vi "ConfDB-GFV.vi"(8 "error in (no error)":errorcluster, 10 "Data in":variant, 11 "Command In":T1=enum."Configure DB") -> (0 "error out":errorcluster, 2 "Data out":variant)   [LabVIEW 2013]
uses:
  ConfEnum.ctl
  ConfDB.ctl
  TypeDef/Magnification.ctl
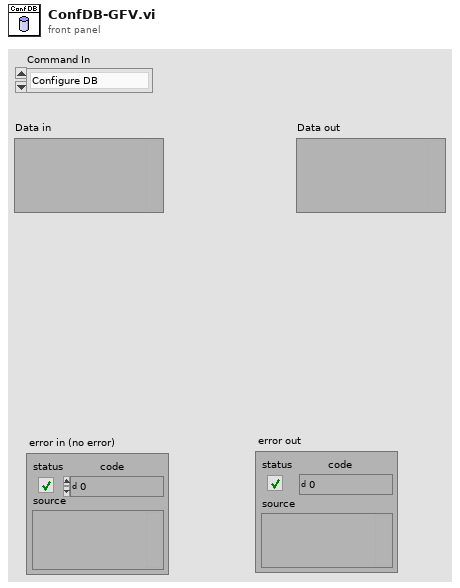
[diagram p1: front panel]
types:
  T1 = typedef "ConfEnum.ctl" = enum16{"Init", "GetConfDB", "GetTemperatureAtIndex", "WriteConfDB", "Configure DB"}
  T2 = typedef "ConfDB.ctl" = cluster{"NumberOfImages":i32, "NoImages2SaveAroundFreeze":i32, "Path":path, "NameOfPartialFile":string, "StartIndex":i32, "NumberOfStdTol":i32, "Detla t (sec)":i32, "Number of images for baseline":i32, "Temperature File Name":string, "Score":dbl, "Index number of Files":i32[], "End Index":i32, "Temperature Array":dbl[], "TStartIndex":i32, "Magnification (Microns/Pixel)":T3, "Circle Descriptor":cluster{"Min Radius":dbl, "Max Radius":dbl}}
  T3 = typedef "Magnification.ctl" = dbl
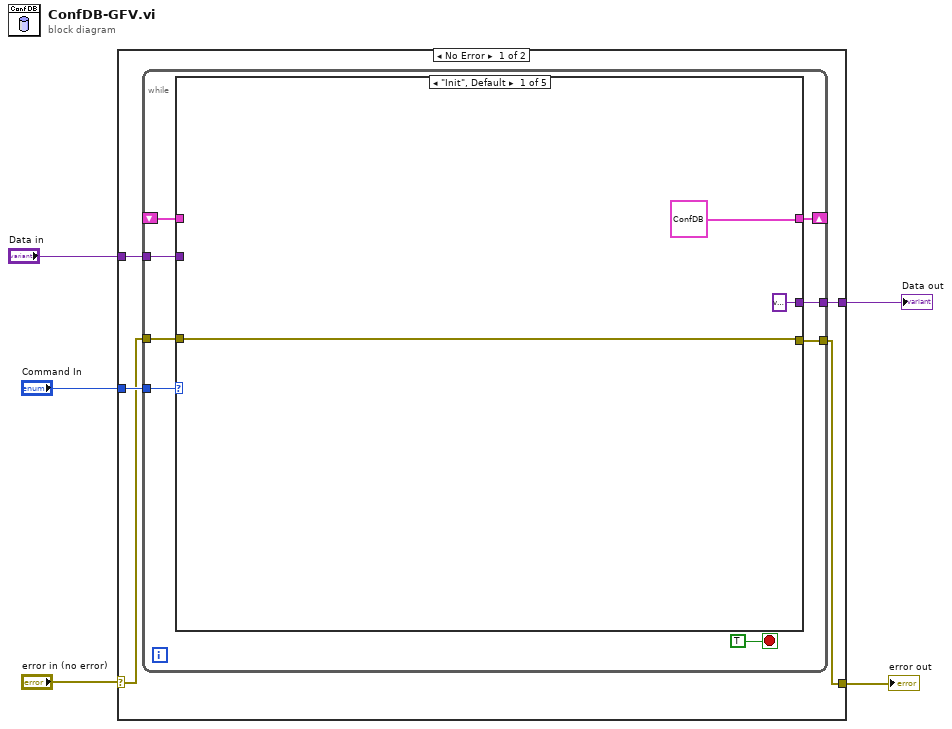
[diagram p0: block diagram]
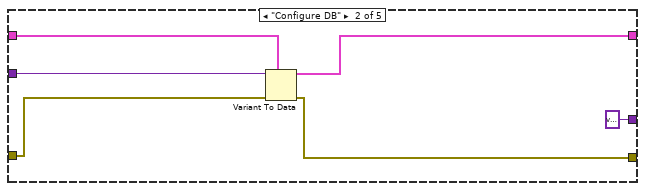
[diagram p2: hidden frame]
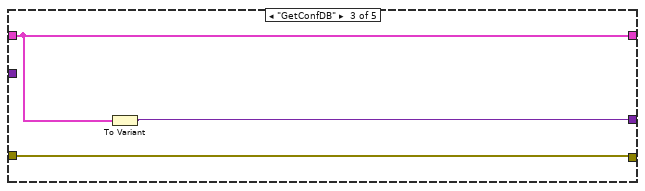
[diagram p3: hidden frame]
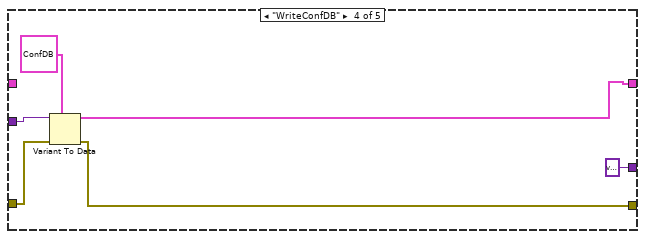
[diagram p4: hidden frame]
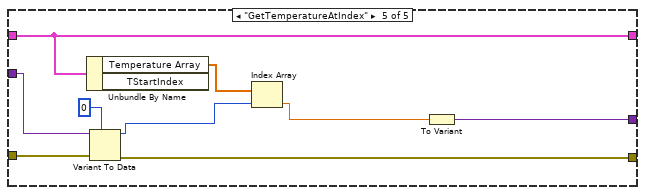
[diagram p5: hidden frame]
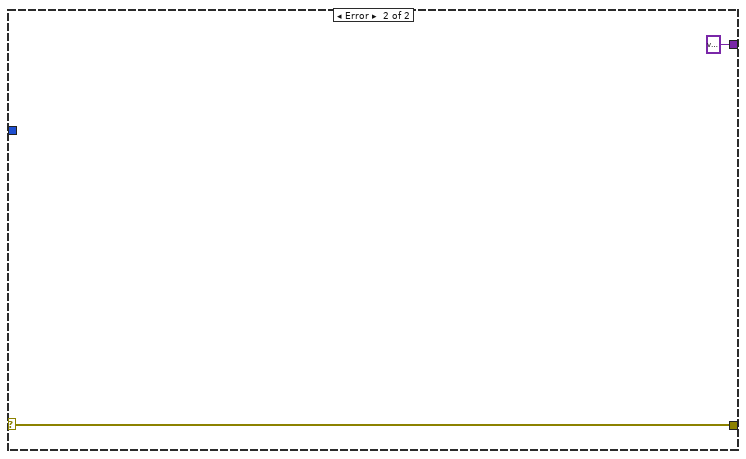
[diagram p6: hidden frame]
diagram:
  n1 = case shown="No Error" "error in (no error)" {
    selector: "error in (no error)" -> [w7 w47]
    tunnel: [w6 w47] -> w4
    tunnel: "Command In" -> [w10 _]
    tunnel: "Data in" -> [w9 _]
    tunnel: [w8 variant ("Variant")] -> w1
    frame No Error {
      n2 = while {
        tunnel: w10 -> [w17]
        shift-right: [w16] -> _
        shift-left: _ -> [w14]
        tunnel: w9 -> [w15]
        tunnel: [w13] -> w8
        tunnel: w7 -> [w12]
        tunnel: [w11] -> w6
        stop <- TRUE stop-if-true
        n3 = case shown="\"Init\", Default" w17 {
          tunnel: [T2 {"NumberOfImages"=0, "NoImages2SaveAroundFreeze"=0, "Path"=path "", "NameOfPartialFile"="", "StartIndex"=0, "NumberOfStdTol"=0, "Detla t (sec)"=0, "Number of images for baseline"=0, "Temperature File Name"="", "Score"=0.0, "Index number of Files"=[], "End Index"=0, "Temperature Array"=[], "TStartIndex"=0, "Magnification (Microns/Pixel)"=0.0, "Circle Descriptor"={"Min Radius"=0.0, "Max Radius"=0.0}} ("ConfDB") w25 w30 w34 w45] -> w16
          tunnel: w15 -> [_ w27 _ w36 w43]
          tunnel: w14 -> [_ w26 w30 _ w45]
          tunnel: [variant ("Variant") variant ("Variant") w29 variant ("Variant") w39] -> w13
          tunnel: w12 -> [w19 w23 w28 w32 w42]
          tunnel: [w19 w22 w28 w31 w38] -> w11
          frame "Init", Default {
          }
          frame "Configure DB" {
            n4 = Variant To Data(error in=w23, type=w26, Variant=w27) -> (data=w25:T2, error out=w22:errorcluster)
          }
          frame "GetConfDB" {
            n5 = To Variant(anything=w30) -> (Variant=w29:variant)
          }
          frame "WriteConfDB" {
            n6 = Variant To Data(error in=w32, type=T2 {"NumberOfImages"=0, "NoImages2SaveAroundFreeze"=0, "Path"=path "", "NameOfPartialFile"="", "StartIndex"=0, "NumberOfStdTol"=0, "Detla t (sec)"=0, "Number of images for baseline"=0, "Temperature File Name"="", "Score"=0.0, "Index number of Files"=[], "End Index"=0, "Temperature Array"=[], "TStartIndex"=0, "Magnification (Microns/Pixel)"=0.0, "Circle Descriptor"={"Min Radius"=0.0, "Max Radius"=0.0}} ("ConfDB"), Variant=w36) -> (data=w34:T2, error out=w31:errorcluster)
          }
          frame "GetTemperatureAtIndex" {
            n7 = Unbundle By Name(w45) -> ("Temperature Array"=w44:dbl[])  [unwired: 1 out]
            n8 = Variant To Data(error in=w42, type=0, Variant=w43) -> (data=w37:i32, error out=w38:errorcluster)
            n9 = Index Array(array=w44, index=w37) -> (element=w40:dbl)
            n10 = To Variant(anything=w40) -> (Variant=w39:variant)
          }
        }
      }
    }
    frame Error {
    }
  }
  "error out" <- w4
  "Data out" <- w1
